vi "0923_1.vi"() -> ()   [LabVIEW 2020]
panel:
  out "Boolean":bool
  out "output cluster":T1
  out "cluster":T1
  in  "String 3":string="김유신"
  in  "Boolean 3":bool
  in  "Numeric 3":dbl
  out "Numeric 2":dbl
  out "String 2":string
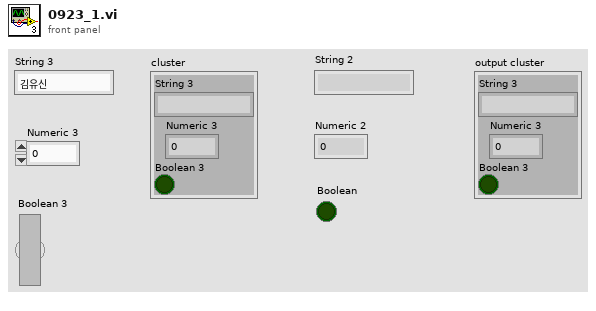
[diagram p1: front panel]
types:
  T1 = cluster{"String 3":string, "Numeric 3":dbl, "Boolean 3":bool}
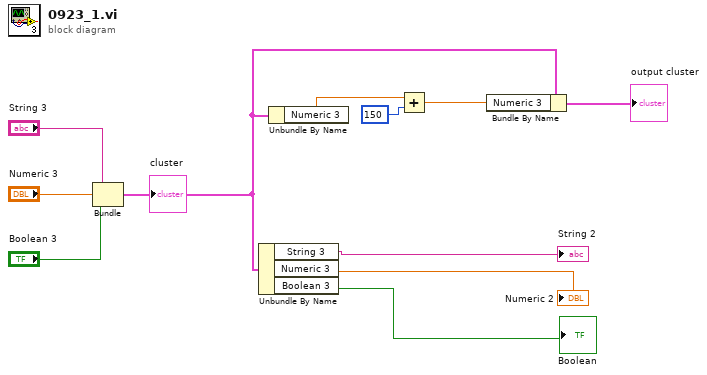
[diagram p0: block diagram]
diagram:
  n1 = Bundle("String 3"="String 3", "Numeric 3"="Numeric 3", "Boolean 3"="Boolean 3") -> (w2:T1)  [unwired: 1 in]
  "cluster" <- w2
  n2 = Unbundle By Name(w2) -> ("String 3"=→"String 2":string, "Numeric 3"=→"Numeric 2":dbl, "Boolean 3"=→"Boolean":bool)
  n3 = Unbundle By Name(w2) -> ("Numeric 3"=w11:dbl)
  n4 = Add(x=w11, y=150) -> (x+y=w9:dbl)
  n5 = Bundle By Name(cluster=w2, "Numeric 3"=w9) -> (→"output cluster":T1)
